vi "Execute Order.vi"(8 "error in (no error)":errorcluster, 11 "Agent in":refnum<class "Agent.lvclass">) -> (0 "error out":errorcluster, 1 "timed out?":bool, 2 "Order Queue":refnum<queue>, 3 "Agent out":refnum<class "Agent.lvclass">)   [LabVIEW 2019, in "Agent.lvclass"]
doc: "Agent (invoker) sends the next order (command) in the order queue to the stock trader for implementation."
uses:
  Agent.lvclass
  Order/Order.lvclass
  Agent.lvclass/Agent.ctl
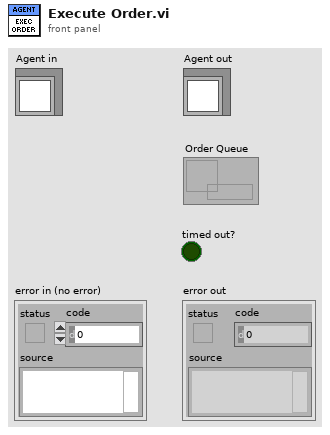
[diagram p1: front panel]
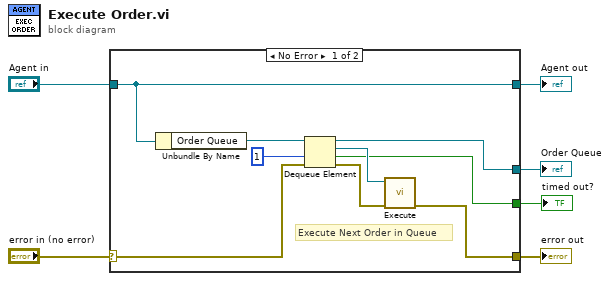
[diagram p0: block diagram]
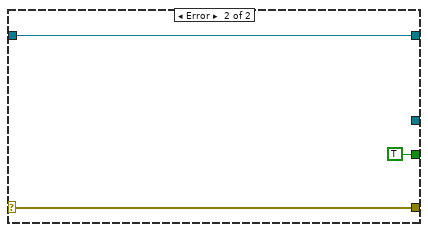
[diagram p2: hidden frame]
diagram:
  n1 = case shown="No Error" "error in (no error)" {
    selector: "error in (no error)" -> [w9 w17]
    tunnel: [w8 w17] -> w5
    tunnel: [w15 w18] -> w3
    tunnel: "Agent in" -> [w15 w18]
    tunnel: [w13 _] -> w2
    tunnel: [w7 TRUE ("timed out?")] -> w1
    frame No Error {
      # "Execute Next Order in Queue"
      n2 = Unbundle By Name(w15) -> ("Order Queue"=w14:refnum<queue>)
      n3 = Dequeue Element(queue=w14, timeout in ms (-1)=1, error in (no error)=w9) -> (queue out=w13:refnum<queue>, element=w11:refnum<class "Order.lvclass">, timed out?=w7:bool, error out=w10:errorcluster)
      n4 = call-dynamic "Execute.vi"("error in (no error)"=w10, "Order In"=w11) -> ("error out"=w8:errorcluster)  [unwired: 8 in, 1 out]
    }
    frame Error {
    }
  }
  "error out" <- w5
  "Agent out" <- w3
  "Order Queue" <- w2
  "timed out?" <- w1
